vi "AiTo32Bit.vi"(1 "AI 0":i16, 2 "AI 1":i16) -> (0 "AI 32bit":u32)   [LabVIEW 2014]
doc: "Converts four I16 int to one I64.\nUsed to bundle 4 analog input samples to one 64 bit input for the DRAM."
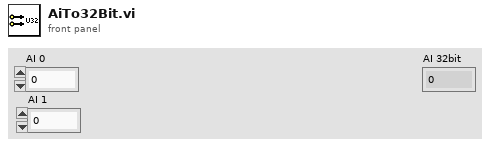
[diagram p1: front panel]
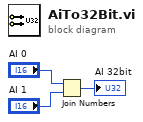
[diagram p0: block diagram]
diagram:
  n1 = Join Numbers(hi="AI 0", lo="AI 1") -> ((hi.lo)=→"AI 32bit":u32)
